vi "Get Deepest Common Directory.vi"(8 "Error In":errorcluster, 11 "File Paths":path[](array[path])) -> (0 "Error Out":errorcluster, 2 "Deepest Common Path":path, 3 "Duplicate File Paths":path[](array[path]))   [LabVIEW 2011, in "LMH-Toolbox.lvlib"]
doc: "Given an array of file paths find the deepest common directory. This is the deepest path that is common to all files specified."
uses:
  LMH-Toolbox.lvlib
panel:
  out "Common Directory Found?":bool
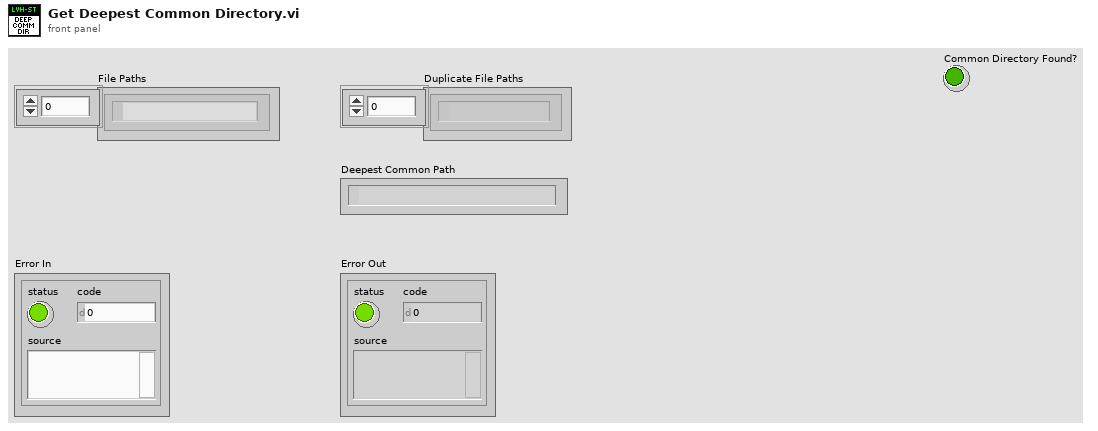
[diagram p1: front panel]
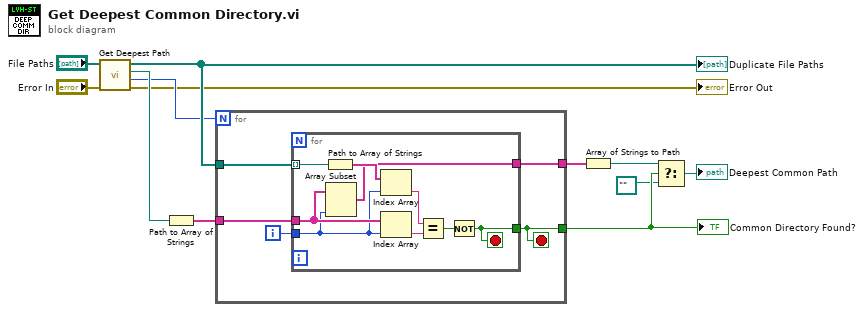
[diagram p0: block diagram]
diagram:
  n1 = call "Get Deepest Path.vi"("Error In"="Error In", "File Paths"="File Paths") -> ("Error Out"=→"Error Out":errorcluster, "Path Tokens"=w8:i32, "Deepest Path"=w11:path, "Duplicate File Paths"=w10:path[])  [unwired: 6 in]
  "Duplicate File Paths" <- w10
  n2 = Path to Array of Strings(0:w11) -> (2:w9:string[])  [unwired: 1 out]
  n3 = for {
    N: w8 -> [_]
    tunnel: w10 -> [w17]
    tunnel: w9 -> [w16]
    tunnel: [w14] -> w4
    tunnel: [w13] -> w1
    i -> [w15]
    stop <- w14 stop-if-true
    n4 = for {
      tunnel: w17 -> [w26] mode=indexing
      tunnel: w16 -> [w21]
      tunnel: w15 -> [w18]
      tunnel: [w20] -> w13
      tunnel: [w19] -> w14
      stop <- w19 stop-if-true
      n5 = Path to Array of Strings(0:w26) -> (2:w25:string[])  [unwired: 1 out]
      n6 = Array Subset(array=w21, length=w18) -> (w20:string[])  [unwired: 1 in]
      n7 = Index Array(array=w25, index=w18) -> (element=w24:string)
      n8 = Index Array(array=w21, index=w18) -> (element=w23:string)
      n9 = Equal?(x=w24, y=w23) -> (x = y?=w22:bool)
      n10 = Not(x=w22) -> (.not. x?=w19:bool)
    }
  }
  "Common Directory Found?" <- w4
  n11 = Array of Strings to Path(0:w1) -> (2:w5:path)  [unwired: 1 in]
  n12 = Select(t=w5, s=w4, f=path "") -> (s? t:f=→"Deepest Common Path":path)
